vi "Predict.vi"(9 "PDP_Array_Data":dbl, 10 "Error_Model_Path":string, 11 "Polarization_Model_Path":string) -> (1 "Predicted Absolute Error":dbl, 2 "Predicted Relative Error":dbl, 3 "Predicted Polarization":dbl)   [LabVIEW 2024]
panel:
  out "error out":errorcluster
  out "session out":refnum<k35>
  in  "error in (no error)":errorcluster
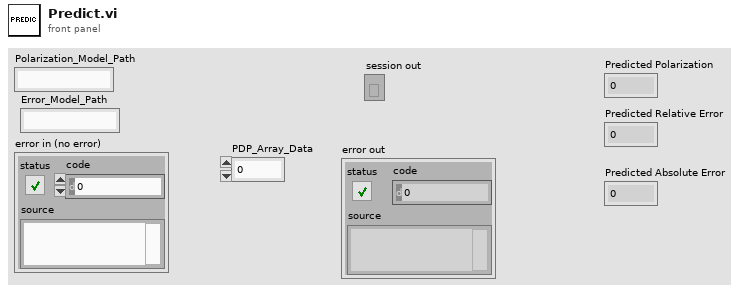
[diagram p1: front panel]
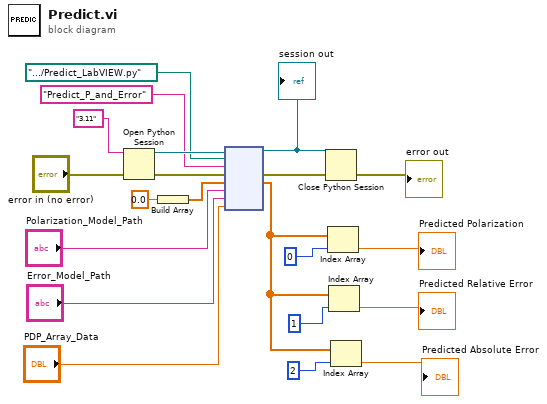
[diagram p0: block diagram]
diagram:
  n1 = Open Python Session(python version="3.11" ("Python version")) -> (session out=w18:refnum<k35>)  [unwired: 2 in, 1 out]
  n2 = Build Array(0.0) -> (w8:dbl[])
  n3 = node(w18, path ".../Predict_LabVIEW.py" ("module path"), "Predict_P_and_Error" ("function name"), "error in (no error)", w8, "Polarization_Model_Path", "Error_Model_Path", "PDP_Array_Data") -> (w13:refnum<k35>, →"error out":errorcluster, w4:dbl[])  [unwired: 3 in, 2 out]
  "session out" <- w13
  n4 = Close Python Session(session in=w13) -> ()  [unwired: 1 in, 1 out]
  n5 = Index Array(array=w4, index=0) -> (element=→"Predicted Polarization":dbl)
  n6 = Index Array(array=w4, index=1) -> (element=→"Predicted Relative Error":dbl)
  n7 = Index Array(array=w4, index=2) -> (element=→"Predicted Absolute Error":dbl)
